vi "Execute.vi"(2 "error in":errorcluster) -> (0 "error out":errorcluster, 1 "Enum":T1(ring)=enum."Initialize")   [LabVIEW 2017]
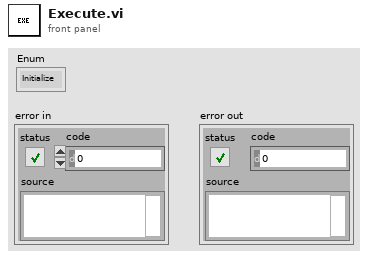
[diagram p1: front panel]
types:
  T1 = enum16{"Terminate", "Finalize", "Execute", "Initialize"}
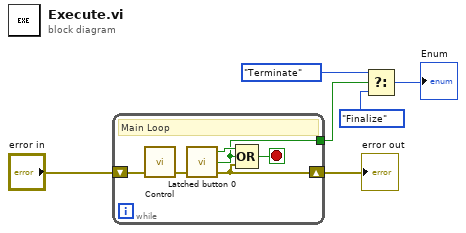
[diagram p0: block diagram]
diagram:
  n1 = while {
    shift-right: [w9] -> w5
    shift-left: "error in" -> [w11]
    tunnel: [w7] -> w6
    stop <- w12 stop-if-true
    # "Main Loop"
    n2 = call "Control.vi"("error in (no error)"=w11) -> ("error out"=w10:errorcluster)  [unwired: 4 in]
    n3 = call "Latched button 0.vi"("error in (no error)"=w10) -> ("error out"=w9:errorcluster, "Long Pressed"=w7:bool, "Latched"=w8:bool)  [unwired: 2 in]
    n4 = Compound Arithmetic op=OR(w8, w7, w9) -> (w12:bool)
  }
  "error out" <- w5
  n5 = Select(t=T1."Terminate", s=w6, f=T1."Finalize") -> (s? t:f=→"Enum":T1)
